vi "LinearPlntInvFF_Reset_Initial.vi"(10 "initialState":T1, 11 "Input Linear Plant Inv FF":T2) -> (3 "Output Linear Plant Inv FF":T2)   [LabVIEW 2019, in "Trajectory_Library.lvlib"]
doc: "Creates a new LINEAR PLANT INVERSION FEEDFORWARD data cluster with the specified values. \n\n\nInputs: \n - XXX -- XXX.\n\nOutputs:\n - XXX -- XXX."
uses:
  Trajectory_Library.lvlib
  LINEAR_PLANT_INV_FF.ctl
  <vilib>/Analysis/Matrix/Datatypes/RealMatrix.ctl
  <vilib>/Analysis/Matrix/NI_Matrix.lvlib
panel:
  # "<States,1>"
  # "<Inputs,1>"
  # "<States,Inputs>"
  # "<States,States>"
  # "<States,1>"
  # "<Inputs,1>"
  # "<States,Inputs>"
  # "<States,States>"
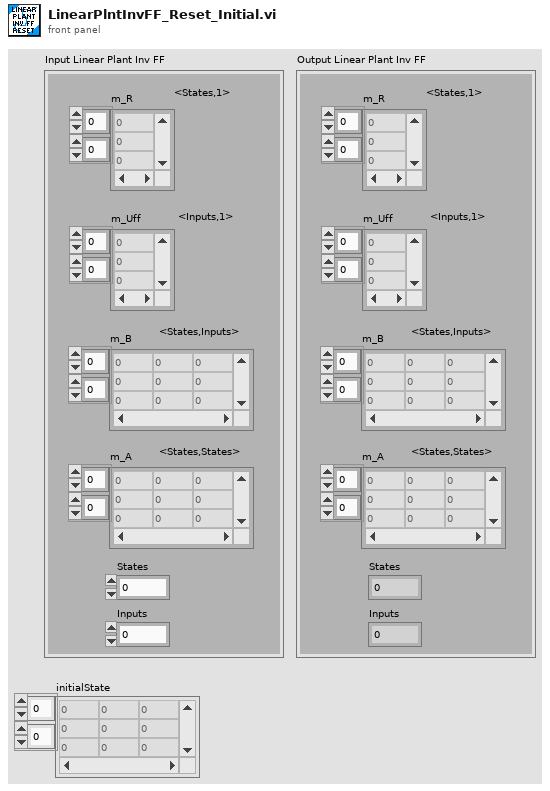
[diagram p1: front panel]
types:
  T1 = typedef "NI_Matrix.lvlib/RealMatrix.ctl" = dbl[][]
  T2 = typedef "Trajectory_Library.lvlib/LINEAR_PLANT_INV_FF.ctl" = cluster{"m_R":T1, "m_Uff":T1, "m_B":T1, "m_A":T1, "States":i32, "Inputs":i32}
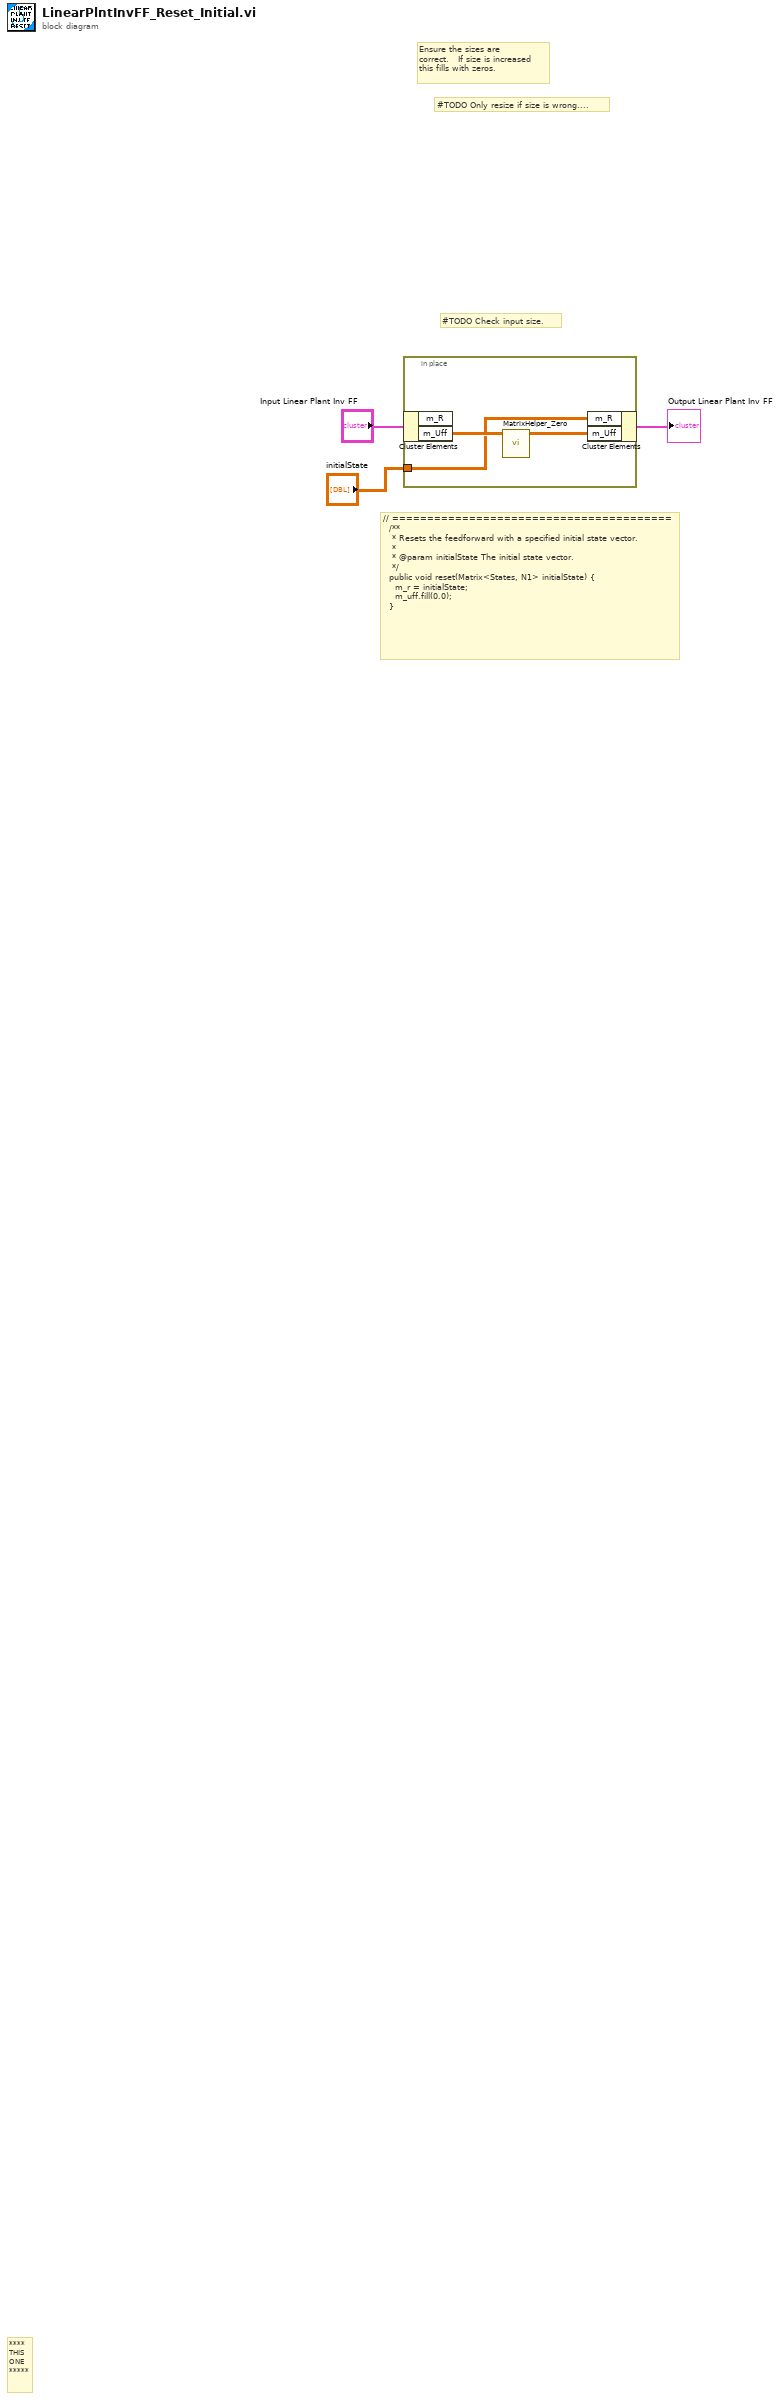
[diagram p0: block diagram]
diagram:
  # "#TODO Check input size."
  # "// ========================================\n  /**\n   * Resets the feedforward with a specified initial state vector.\n   *\n   * @param initialState The initial state vector.\n   */\n  public void reset(Matrix<States, N1> initialState) {\n    m_r = initialState;\n    m_uff.fill(0.0);\n  }"
  # "#TODO Only resize if size is wrong...."
  # "Ensure the sizes are\ncorrect.   If size is increased \nthis fills with zeros."
  # "****\nTHIS\nONE\n*****"
  n1 = in-place {
    in-place-border: "initialState" -> [w4]
    n2 = in-place-cluster #1("Input Linear Plant Inv FF") -> ("m_Uff"=w6:T1)  [unwired: 1 out]
    n3 = call "MatrixHelper_Zero.vi"("input matrix"=w6) -> ("output matrix"=w5:T1)  [unwired: 10 in]
    n4 = in-place-cluster #1("m_R"=w4, "m_Uff"=w5) -> (→"Output Linear Plant Inv FF":T2)
  }
